vi "setup.vi"() -> (2 "delay, begin, stop settings 2":dbl[](array[numeric]), 3 "Keithley 6431":bool, 4 "J-KEM2":bool, 6 "Keithley 2421":bool, 8 "SRS QCM 2":bool, 10 "error IO":errorcluster, 12 "Arduino2":bool, 13 "Auto Stop 2":bool, 14 "Pressure control 2":bool, 15 "Save file path 2":path)   [LabVIEW 2014]
panel:
  in  "Save file path":path
  in  "Pressure control":bool
  in  "J-KEM":bool
  in  "Arduino":bool
  in  "Keithley 6430":bool
  in  "Keithley 2420":bool
  in  "Auto stop after":bool
  in  "delay, begin, stop settings":dbl[](array[numeric]) caption="Delay betwen data points (s)\n\nBegin recording data after (min)\n\nAuto stop after (hrs)"
  in  "SRS QCM":bool
  in  "OK":bool
  # "Instruments Connected"
  # "Manual timing settings"
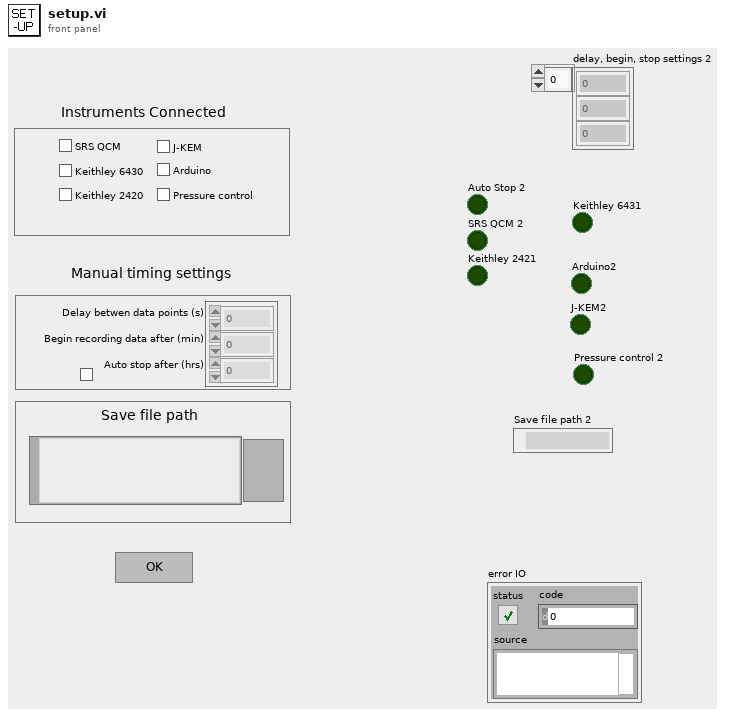
[diagram p1: front panel]
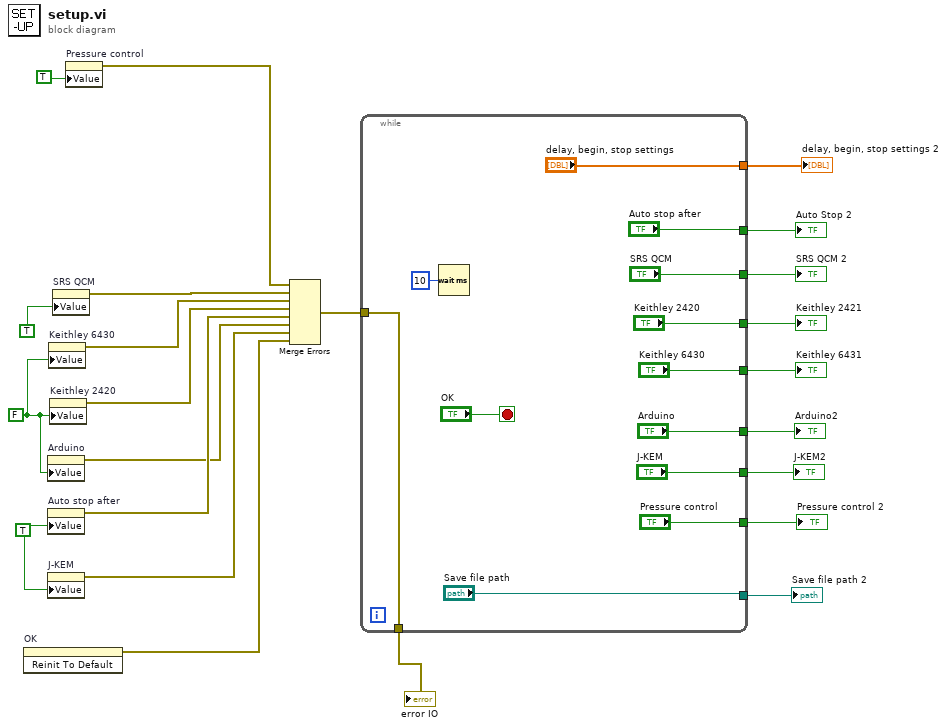
[diagram p0: block diagram]
diagram:
  w5 = TRUE ("Auto Stop")
  w3 = FALSE ("Auto Stop")
  n1 = invoke on="OK" class="Bool" method="Reinit To Default"() -> (error out=w17:errorcluster)  [unwired: 3 in, 2 out]
  n2 = property on="Arduino" class="Bool (strict)"("Value"=w3) -> (error out=w11:errorcluster)  [unwired: 2 in, 1 out]
  n3 = property on="Auto stop after" class="Bool (strict)"("Value"=w5) -> (error out=w16:errorcluster)  [unwired: 2 in, 1 out]
  n4 = property on="J-KEM" class="Bool (strict)"("Value"=w5) -> (error out=w9:errorcluster)  [unwired: 2 in, 1 out]
  n5 = property on="Keithley 6430" class="Bool (strict)"("Value"=w3) -> (error out=w13:errorcluster)  [unwired: 2 in, 1 out]
  n6 = property on="Keithley 2420" class="Bool (strict)"("Value"=w3) -> (error out=w15:errorcluster)  [unwired: 2 in, 1 out]
  n7 = property on="SRS QCM" class="Bool (strict)"("Value"=TRUE ("Auto Stop")) -> (error out=w12:errorcluster)  [unwired: 2 in, 1 out]
  n8 = property on="Pressure control" class="Bool (strict)"("Value"=TRUE ("Auto Stop")) -> (error out=w1:errorcluster)  [unwired: 2 in, 1 out]
  n9 = Merge Errors(w1, w12, w13, w15, w16, w11, w9, w17) -> (w23:errorcluster)
  n10 = while {
    tunnel: w23 -> [w25]
    tunnel: ["SRS QCM"] -> w21
    tunnel: ["Auto stop after"] -> w22
    tunnel: ["Keithley 2420"] -> w20
    tunnel: ["Keithley 6430"] -> w19
    tunnel: ["Arduino"] -> w18
    tunnel: ["J-KEM"] -> w10
    tunnel: ["Pressure control"] -> w7
    tunnel: ["Save file path"] -> w6
    tunnel: [w25] -> w4
    tunnel: ["delay, begin, stop settings"] -> w2
    stop <- "OK" stop-if-true
    n11 = Wait (ms)(milliseconds to wait=u32 10) -> ()  [unwired: 1 out]
  }
  "Auto Stop 2" <- w22
  "SRS QCM 2" <- w21
  "Keithley 2421" <- w20
  "Keithley 6431" <- w19
  "Arduino2" <- w18
  "J-KEM2" <- w10
  "Pressure control 2" <- w7
  "Save file path 2" <- w6
  "error IO" <- w4
  "delay, begin, stop settings 2" <- w2
